vi "Create Types.vi"(8 "error in (no error)":errorcluster, 11 "protoFile ref in":u64) -> (0 "error out":errorcluster, 2 "Enum Parameters":T1[](array[typedef]), 3 "Message Parameters":T2[](array[typedef]))   [LabVIEW 2019, in "gRPC Template Creation Utility.lvlib"]
uses:
  gRPC Template Creation Utility.lvlib
  TypeDefs/Message Metadata (Scripting).ctl
  TypeDefs/Message Element Metadata (Scripting).ctl
  TypeDefs/Message Element Type.ctl
  TypeDefs/Enum Metadata (Scripting).ctl
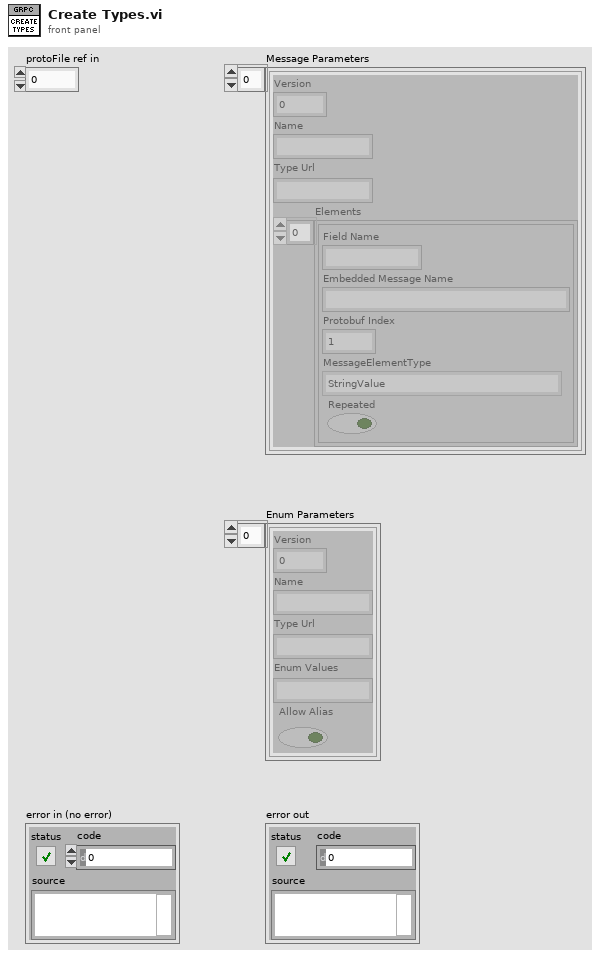
[diagram p1: front panel]
types:
  T1 = typedef "gRPC Template Creation Utility.lvlib/Enum Metadata (Scripting).ctl" = cluster{"Version":i32, "Name":string, "Type Url":string, "Enum Values":string, "Allow Alias":bool}
  T2 = typedef "gRPC Template Creation Utility.lvlib/Message Metadata (Scripting).ctl" = cluster{"Version":i32, "Name":string, "Type Url":string, "Elements":T3[]}
  T3 = typedef "gRPC Template Creation Utility.lvlib/Message Element Metadata (Scripting).ctl" = cluster{"Field Name":string, "Embedded Message Name":string, "Protobuf Index":i32, "MessageElementType":T4, "Repeated":bool}
  T4 = typedef "gRPC Template Creation Utility.lvlib/Message Element Type.ctl" = enum32{"Int32Value", "FloatValue", "DoubleValue", "BoolValue", "StringValue", "MessageValue", "Int64Value", "UInt32Value", "UInt64Value", "EnumValue", "Bytes", "Fixed64", "Fixed32", "SFixed64", "SFixed32", "SInt64", "SInt32"}
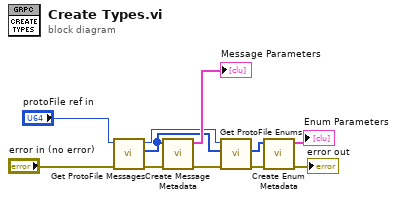
[diagram p0: block diagram]
diagram:
  n1 = call "Get ProtoFile Messages.vi"("error in (no error)"="error in (no error)", "Protofile ref in"="protoFile ref in") -> ("error out"=w4:errorcluster, "ProtoFile Messages"=w8:u64[], "Protofile ref out"=w7:u64)  [unwired: 7 in]
  n2 = call "Create Message Metadata.vi"("error in (no error)"=w4, "ProtoFile Messages"=w8) -> ("error out"=w2:errorcluster, "Message Parameters"=→"Message Parameters":T2[])  [unwired: 8 in]
  n3 = call "Get ProtoFile Enums.vi"("error in (no error)"=w2, "ProtoFile Messages"=w8, "Protofile ref in"=w7) -> ("error out"=w3:errorcluster, "ProtoFile Enums"=w10:u64[])  [unwired: 6 in, 1 out]
  n4 = call "Create Enum Metadata.vi"("error in (no error)"=w3, "ProtoFile Enums"=w10) -> ("error out"=→"error out":errorcluster, "Enum Parameters"=→"Enum Parameters":T1[])  [unwired: 8 in]
